vi "search4obj.vi"(7 "raw dxf in":string) -> (0 "deafult obj properies of interest":string[](array[string]), 3 "obj found?":bool, 4 "found dxf obj raw":string, 5 "raw dxf minus object found":string)   [LabVIEW 2016, in "Dxf.lvlib"]
uses:
  Dxf.lvlib
  <vilib>/regexp/Match Regular Expression.xnode
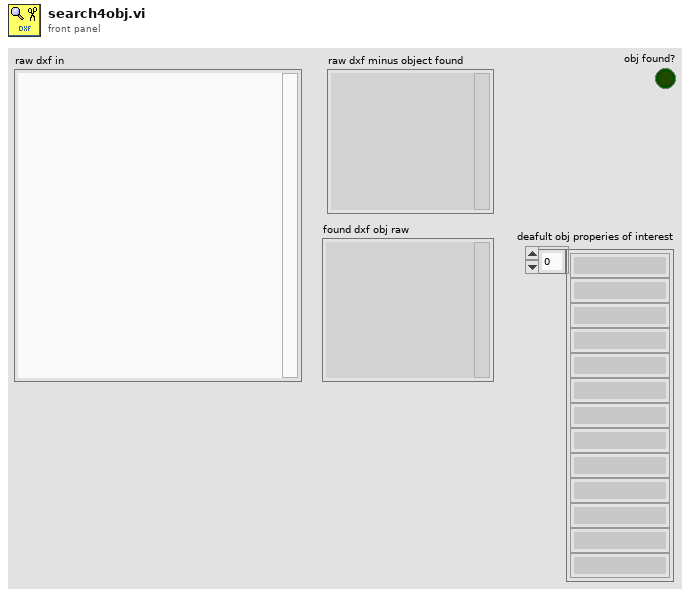
[diagram p1: front panel]
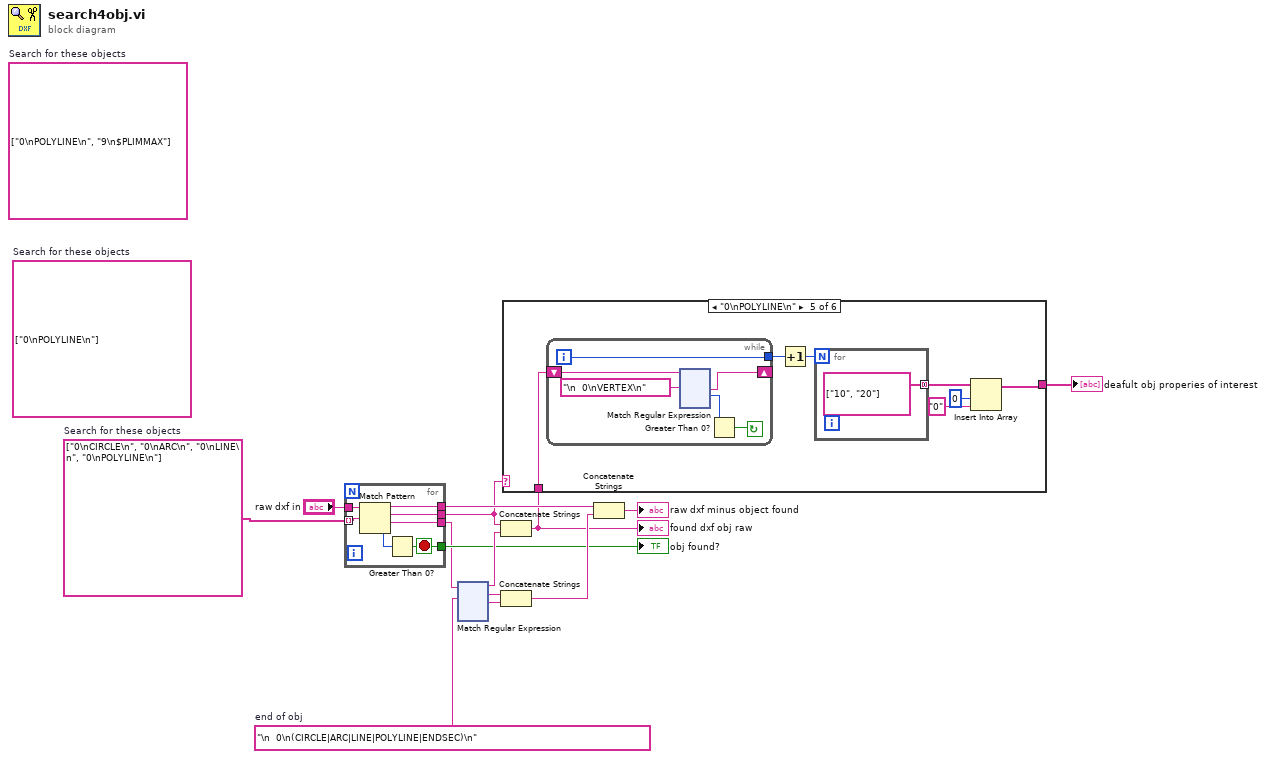
[diagram p0: block diagram]
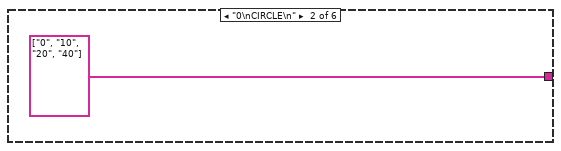
[diagram p3: hidden frame]
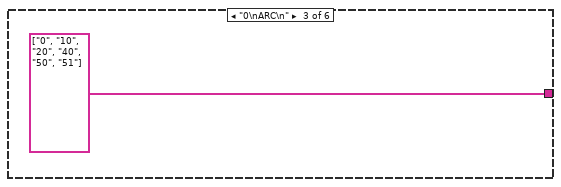
[diagram p4: hidden frame]
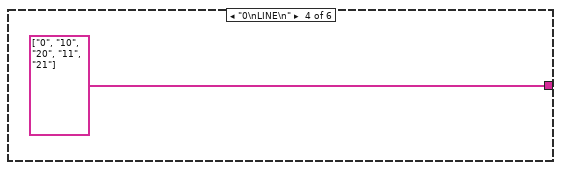
[diagram p5: hidden frame]
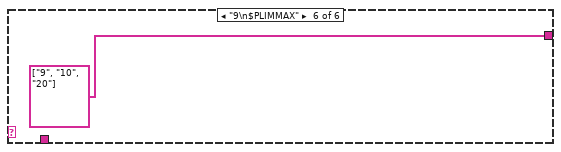
[diagram p6: hidden frame]
diagram:
  (unwired) string[] ["0\nPOLYLINE\n", "9\n$PLIMMAX"]  # Search for these objects
  (unwired) string[] ["0\nPOLYLINE\n"]  # Search for these objects
  w2 = string[] ["0\nCIRCLE\n", "0\nARC\n", "0\nLINE\n", "0\nPOLYLINE\n"]  # Search for these objects
  w4 = "\n  0\n(CIRCLE|ARC|LINE|POLYLINE|ENDSEC)\n"  # end of obj
  n1 = for {
    tunnel: [w19] -> w5
    tunnel: [w20] -> w3
    tunnel: [w18] -> w7
    tunnel: "raw dxf in" -> [w17]
    tunnel: [w16] -> w11
    tunnel: w2 -> [w15] mode=indexing
    stop <- w19 stop-if-true
    n2 = Match Pattern(string=w17, regular expression=w15) -> (before substring=w16:string, match substring=w18:string, after substring=w20:string, offset past match=w21:i32)  [unwired: 1 in]
    n3 = Greater Than 0?(x=w21) -> (x > 0?=w19:bool)
  }
  "obj found?" <- w5
  n4 = xnode "Match Regular Expression"("input string"=w3, "regular expression"=w4) -> ("before match"=w10:string, "whole match"=w9:string, "after match"=w8:string)  [unwired: 4 in, 2 out]
  n5 = Concatenate Strings(w7, w10) -> (w1:string)
  "found dxf obj raw" <- w1
  n6 = Concatenate Strings(w9, w8) -> (w12:string)
  n7 = case shown="\"0\\nPOLYLINE\\n\"" w7 {
    tunnel: [_ string[] ["0", "10", "20", "40"] string[] ["0", "10", "20", "40", "50", "51"] string[] ["0", "10", "20", "11", "21"] w27 string[] ["9", "10", "20"]] -> w6
    tunnel: w1 -> [_ _ _ _ w31 _]
    frame Default {
    }
    frame "0\nCIRCLE\n" {
    }
    frame "0\nARC\n" {
    }
    frame "0\nLINE\n" {
    }
    frame "0\nPOLYLINE\n" {
      n8 = while {
        shift-right: [w36] -> _
        shift-left: w31 -> [w37]
        tunnel: [w34] -> w30
        i -> [w34]
        stop <- w32 continue-if-true
        n9 = xnode "Match Regular Expression"("input string"=w37, "regular expression"="\n  0\nVERTEX\n") -> ("after match"=w36:string, "offset past match"=w33:i32)  [unwired: 4 in, 3 out]
        n10 = Greater Than 0?(x=w33) -> (x > 0?=w32:bool)
      }
      n11 = Increment(x=w30) -> (x+1=w29:i32)
      n12 = for {
        N: w29 -> [_]
        tunnel: [string[] ["10", "20"]] -> w28 mode=concatenating
      }
      n13 = Insert Into Array(array=w28, index=0, new element="0" ("new element/subarray")) -> (w27:string[])
    }
    frame "9\n$PLIMMAX" {
    }
  }
  "deafult obj properies of interest" <- w6
  n14 = Concatenate Strings(w11, w12) -> (→"raw dxf minus object found":string)
